vi "LS2.vi"(0 "LS1":bool, 7 "LS3":bool, 9 "LS4":bool, 11 "LS5":bool) -> (6 "State Selector":T1)   [LabVIEW 2017]
uses:
  state_R.ctl
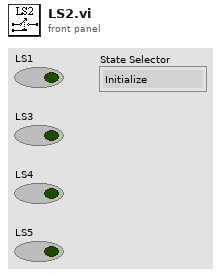
[diagram p1: front panel]
types:
  T1 = typedef "state_R.ctl" = enum16{"Initialize", "State 1", "State 2", "State 3", "State 4", "State 5", "State 6", "State 7", "State 8", "State 9", "UP", "DOWN", "EXTEND", "BACK", "Reset", "Process", "PAUSE", "Report", "Halt", "Shutdown"}
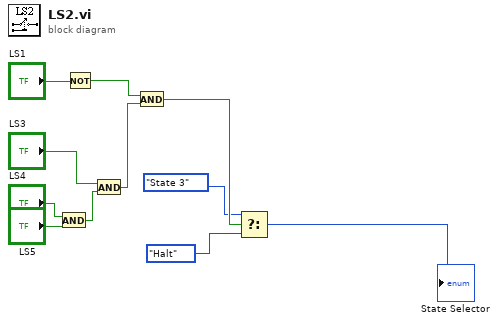
[diagram p0: block diagram]
diagram:
  n1 = And(x="LS4", y="LS5") -> (x .and. y?=w2:bool)
  n2 = Not(x="LS1") -> (.not. x?=w4:bool)
  n3 = And(x="LS3", y=w2) -> (x .and. y?=w3:bool)
  n4 = And(x=w4, y=w3) -> (x .and. y?=w5:bool)
  n5 = Select(t=state_R."State 3" ("State Selector"), s=w5, f=state_R."Halt" ("State Selector")) -> (s? t:f=→"State Selector":T1)
